vi "rotation matrix.vi"(2 "angle":dbl, 3 "y":dbl, 4 "x":dbl) -> (0 "new y":dbl, 1 "new x":dbl)   [LabVIEW 2021]
doc: "Rotation matrix"
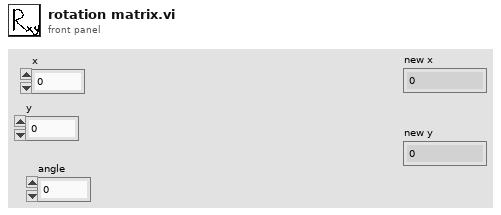
[diagram p1: front panel]
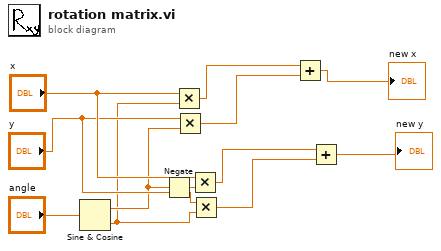
[diagram p0: block diagram]
diagram:
  n1 = Sine & Cosine(0:"angle") -> (1:w4:dbl, 2:w2:dbl)
  n2 = Negate(x=w4) -> (-x=w3:dbl)
  n3 = Multiply(x="x", y=w2) -> (x*y=w10:dbl)
  n4 = Multiply(x="y", y=w4) -> (x*y=w9:dbl)
  n5 = Multiply(x="x", y=w3) -> (x*y=w8:dbl)
  n6 = Multiply(x="y", y=w2) -> (x*y=w7:dbl)
  n7 = Add(x=w10, y=w9) -> (x+y=→"new x":dbl)
  n8 = Add(x=w8, y=w7) -> (x+y=→"new y":dbl)
